vi "Configure Offset and Limits (Demodulation - ASK).vi"(0 "VISA resource name":refnum<visa-resource-name>, 1 "ASK Depth Upper (90 percentage)":dbl=90.0, 3 "Carrier Frequency Offset Upper (1E+6 Hz)":dbl=1000000.0, 5 "Enable Limit (F: Disable)":bool, 9 "Carrier Power Upper (10 dBm)":dbl=10.0, 11 "error in (no error)":errorcluster, 12 "ASK Depth Lower (0.1 percentage)":dbl=0.1) -> (4 "VISA resource name out":refnum<visa-resource-name>, 15 "error out":errorcluster)   [LabVIEW 2022 SP3, in "Agilent N934X Series.lvlib"]
doc: "Configures the general setting for ASK demodulation offset and limits of Demodulation Option.\n\nNote:\nThis VI is only applicable for N9321C, N9322C, N9323C, N9324C models."
uses:
  <instrlib>/Agilent N934X Series/Agilent N934X Series.lvlib
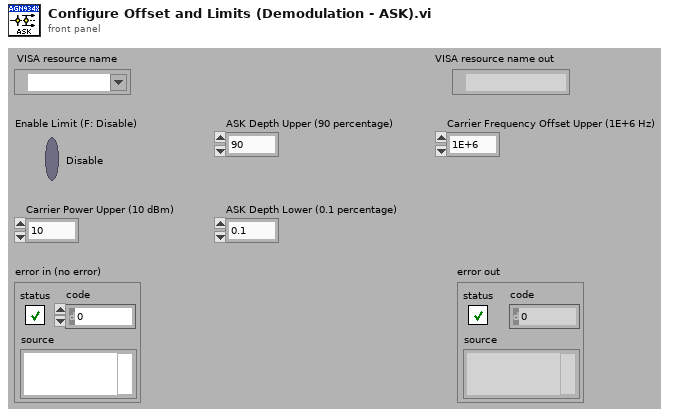
[diagram p1: front panel]
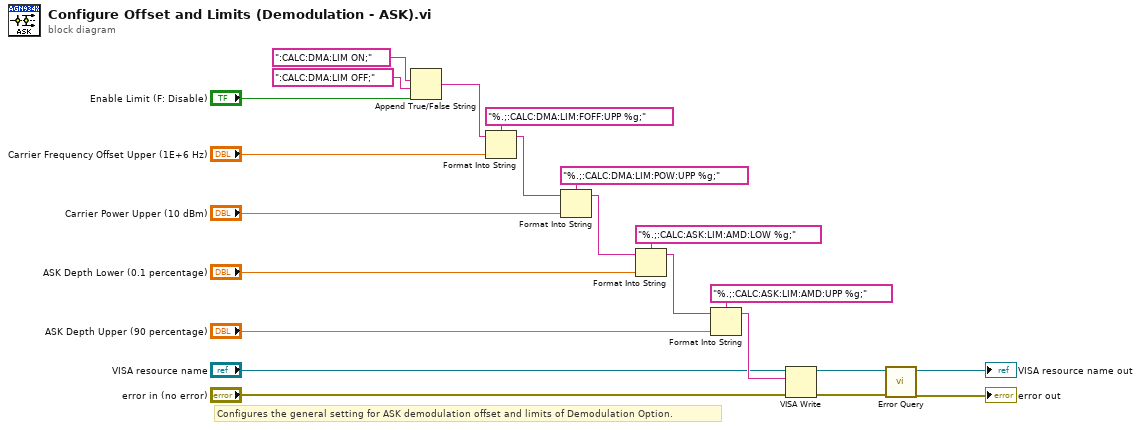
[diagram p0: block diagram]
diagram:
  # "Configures the general setting for ASK demodulation offset and limits of Demodulation Option."
  n1 = Append True/False String(1:"Enable Limit (F: Disable)", 2:":CALC:DMA:LIM OFF;", 3:":CALC:DMA:LIM ON;") -> (0:w19:string)  [unwired: 1 in]
  n2 = Format Into String(format string="%.;:CALC:DMA:LIM:FOFF:UPP %g;", initial string=w19, "Carrier Frequency Offset Upper (1E+6 Hz)") -> (resulting string=w16:string)  [unwired: 1 in, 1 out]
  n3 = Format Into String(format string="%.;:CALC:DMA:LIM:POW:UPP %g;", initial string=w16, "Carrier Power Upper (10 dBm)") -> (resulting string=w13:string)  [unwired: 1 in, 1 out]
  n4 = Format Into String(format string="%.;:CALC:ASK:LIM:AMD:LOW %g;", initial string=w13, "ASK Depth Lower (0.1 percentage)") -> (resulting string=w10:string)  [unwired: 1 in, 1 out]
  n5 = Format Into String(format string="%.;:CALC:ASK:LIM:AMD:UPP %g;", initial string=w10, "ASK Depth Upper (90 percentage)") -> (resulting string=w7:string)  [unwired: 1 in, 1 out]
  n6 = VISA Write(VISA resource name="VISA resource name", write buffer=w7, error in (no error)="error in (no error)") -> (VISA resource name out=w4:refnum<visa-resource-name>, error out=w3:errorcluster)  [unwired: 1 out]
  n7 = call <instrlib>:"Error Query.vi"("error in (no error)"=w3, "VISA resource name"=w4) -> ("error out"=→"error out":errorcluster, "VISA resource name out"=→"VISA resource name out":refnum<visa-resource-name>)  [unwired: 6 in, 2 out]
